vi "Get Type.vi"(11 "_Rename in":refnum<class "_Rename.lvclass">) -> (2 "Type":string)   [LabVIEW 2021, in "_Rename.lvlib" / "_Rename.lvclass"]
uses:
  _Rename.lvclass
  _Rename.lvclass/_Rename.ctl
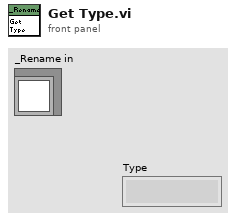
[diagram p1: front panel]
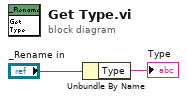
[diagram p0: block diagram]
diagram:
  n1 = Unbundle By Name("_Rename in") -> ("Type"=→"Type":string)
